vi "Set Config.vi"(8 "error in (no error)":errorcluster, 9 "Config Data":variant, 11 "AD4212C in":refnum<class "AD4212C.lvclass">) -> (0 "error out":errorcluster, 3 "AD4212C out":refnum<class "AD4212C.lvclass">)   [LabVIEW 2014, in "AD4212C.lvlib" / "AD4212C.lvclass"]
uses:
  AD4212C.lvclass
  AD4212C.lvclass/AD4212C.ctl
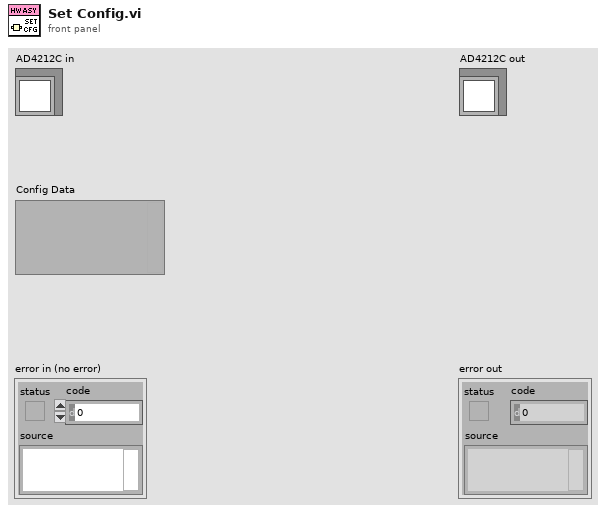
[diagram p1: front panel]
types:
  T1 = typedef "AD4212C Lib.lvlib/Connection Data.ctl" = cluster{"Conection Data":refnum<visa-resource-name>}
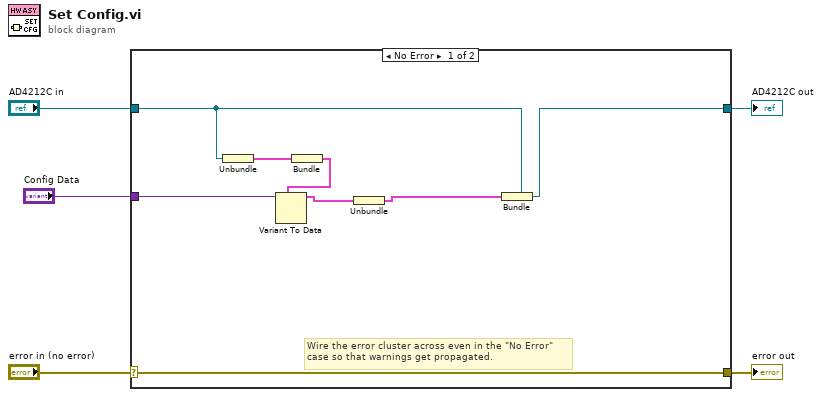
[diagram p0: block diagram]
diagram:
  n1 = case shown="No Error" "error in (no error)" {
    selector: "error in (no error)" -> [w13 w15]
    tunnel: [w13 w15] -> w4
    tunnel: [w11 w14] -> w2
    tunnel: "AD4212C in" -> [w10 w14]
    tunnel: "Config Data" -> [w12 _]
    frame No Error {
      # "Wire the error cluster across even in the \"No Error\"\ncase so that warnings get propagated."
      n2 = Unbundle(w10) -> (w9:T1)
      n3 = Bundle("Connection Data"=w9) -> (w8:cluster{"Connection Data":T1})  [unwired: 1 in]
      n4 = Variant To Data(type=w8, Variant=w12) -> (data=w7:cluster{"Connection Data":T1})  [unwired: 1 in, 1 out]
      n5 = Unbundle(w7) -> ("Connection Data"=w6:T1)
      n6 = Bundle(cluster=w10, w6) -> (w11:refnum<class "AD4212C.lvclass">)
    }
    frame Error {
    }
  }
  "error out" <- w4
  "AD4212C out" <- w2
